vi "AdvanceWaveformPart.vi"(6 "FPGA Cycle Parameters":T1, 7 "FPGA Cycle Counters In":T2, 8 "FPGA Scan Counters In":T3 {"Current part of waveform" items=["Imaging", "Settling", "Resting"]}) -> (1 "Multiplier advance per cycle":fxp<+/-,32,0>, 2 "FPGA Cycle Counters Out":T2, 3 "FPGA Scan Counters Out":T3 {"Current part of waveform" items=["Imaging", "Settling", "Resting"]})   [LabVIEW 2010]
uses:
  FPGA_Typedefs/FPGA Scan Counters.ctl
  FPGA_Typedefs/FPGA Cycle Counters.ctl
  FPGA_Typedefs/FPGA Cycle Parameters.ctl
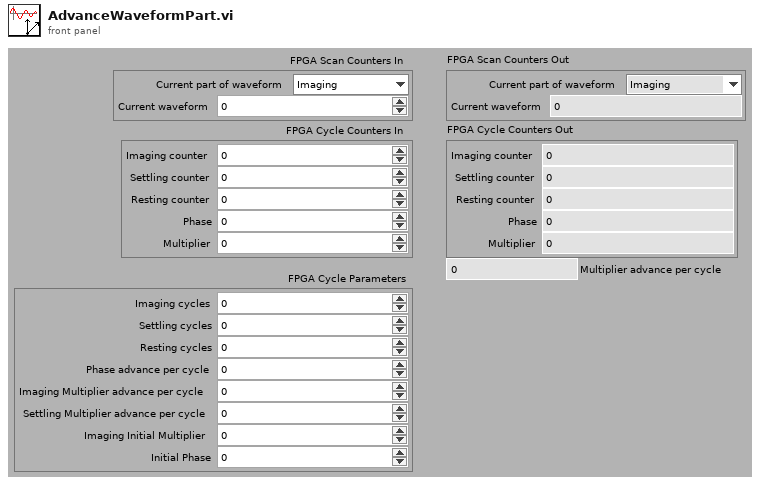
[diagram p1: front panel]
types:
  T1 = typedef "FPGA Cycle Parameters.ctl" = cluster{"Imaging cycles":i32, "Settling cycles":i32, "Resting cycles":i32, "Phase advance per cycle":fxp<+,32,0>, "Imaging Multiplier advance per cycle":fxp<+/-,32,0>, "Settling Multiplier advance per cycle":fxp<+/-,32,0>, "Imaging Initial Multiplier":fxp<+/-,43,12>, "Initial Phase":fxp<+,32,1>}
  T2 = typedef "FPGA Cycle Counters.ctl" = cluster{"Imaging counter":i32, "Settling counter":i32, "Resting counter":i32, "Phase":fxp<+,32,1>, "Multiplier":fxp<+/-,43,12>}
  T3 = typedef "FPGA Scan Counters.ctl" = cluster{"Current part of waveform":u8, "Current waveform":u16}
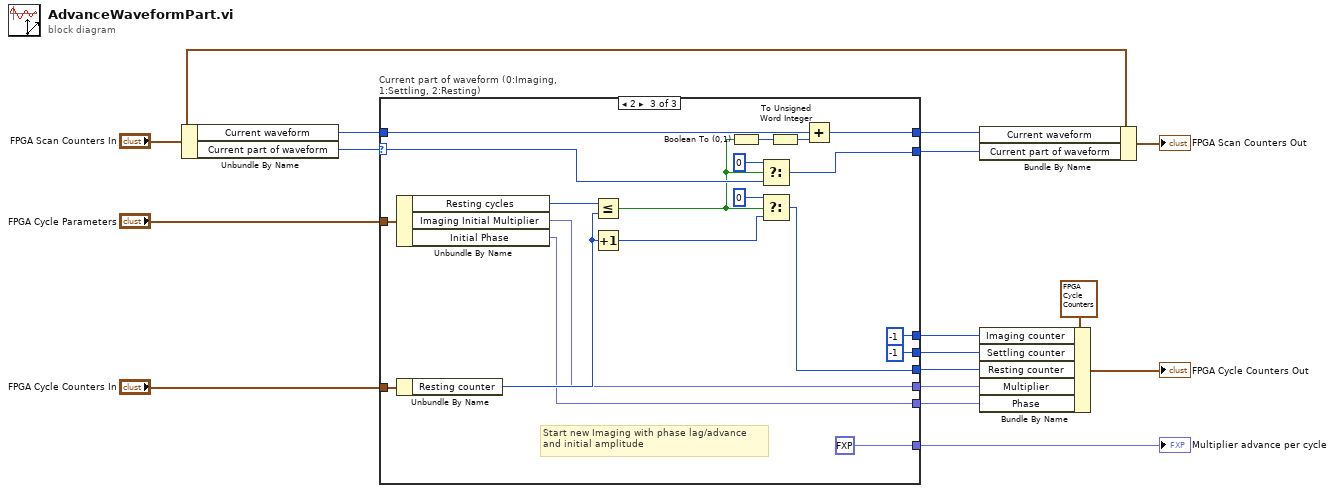
[diagram p0: block diagram]
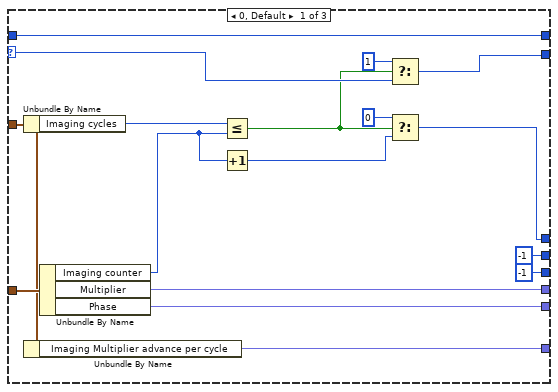
[diagram p2: hidden frame]
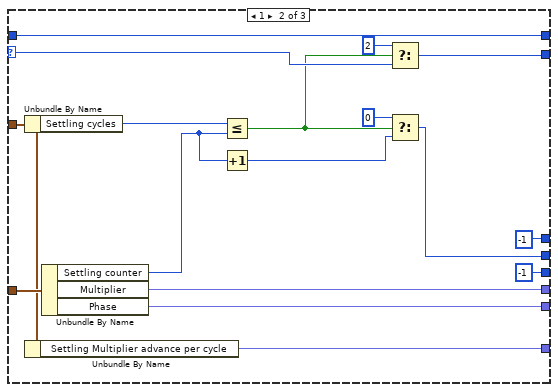
[diagram p3: hidden frame]
diagram:
  n1 = Unbundle By Name("FPGA Scan Counters In") -> ("Current waveform"=w16:u16, "Current part of waveform"=w15:u8)
  n2 = case "Current part of waveform (0:Imaging, 1:Settling, 2:Resting)" shown="2" w15 {
    selector: w15 -> [w33 w49 w69]
    tunnel: [w31 w48 w68] -> w13
    tunnel: w16 -> [w30 w47 w67]
    tunnel: [w30 w47 w66] -> w14
    tunnel: "FPGA Cycle Parameters" -> [w22 w39 w63]
    tunnel: "FPGA Cycle Counters In" -> [w29 w41 w62]
    tunnel: [w28 w43 w58] -> w11
    tunnel: [w24 w42 w57] -> w10
    tunnel: [w21 w38 fxp<+/-,32,0> 0.0 ("Settling Multiplier advance per cycle")] -> w5
    tunnel: [w17 -1 ("Imaging counter") -1 ("Imaging counter")] -> w3
    tunnel: [-1 ("t") w34 -1 ("t")] -> w2
    tunnel: [-1 ("t") -1 ("t") w53] -> w1
    frame 0, Default {
      n3 = Unbundle By Name(w22) -> ("Imaging cycles"=w27:i32)
      n4 = Unbundle By Name(w22) -> ("Imaging Multiplier advance per cycle"=w21:fxp<+/-,32,0>)
      n5 = Unbundle By Name(w29) -> ("Imaging counter"=w20:i32, "Multiplier"=w28:fxp<+/-,43,12>, "Phase"=w24:fxp<+,32,1>)
      n6 = Less Or Equal?(x=w27, y=w20) -> (x <= y?=w23:bool)
      n7 = Increment(x=w20) -> (x+1=w26:i32)
      n8 = Select(t=u8 1, s=w23, f=w33) -> (s? t:f=w31:u8)
      n9 = Select(t=0, s=w23, f=w26) -> (s? t:f=w17:i32)
    }
    frame 1 {
      n10 = Unbundle By Name(w39) -> ("Settling cycles"=w46:i32)
      n11 = Unbundle By Name(w39) -> ("Settling Multiplier advance per cycle"=w38:fxp<+/-,32,0>)
      n12 = Unbundle By Name(w41) -> ("Settling counter"=w37:i32, "Multiplier"=w43:fxp<+/-,43,12>, "Phase"=w42:fxp<+,32,1>)
      n13 = Less Or Equal?(x=w46, y=w37) -> (x <= y?=w40:bool)
      n14 = Increment(x=w37) -> (x+1=w45:i32)
      n15 = Select(t=u8 2, s=w40, f=w49) -> (s? t:f=w48:u8)
      n16 = Select(t=0, s=w40, f=w45) -> (s? t:f=w34:i32)
    }
    frame 2 {
      # "Start new Imaging with phase lag/advance\nand initial amplitude"
      n17 = Unbundle By Name(w63) -> ("Resting cycles"=w65:i32, "Imaging Initial Multiplier"=w58:fxp<+/-,43,12>, "Initial Phase"=w57:fxp<+,32,1>)
      n18 = Unbundle By Name(w62) -> ("Resting counter"=w61:i32)
      n19 = Less Or Equal?(x=w65, y=w61) -> (x <= y?=w60:bool)
      n20 = Increment(x=w61) -> (x+1=w54:i32)
      n21 = Boolean To (0,1)(Boolean=w60) -> (0, 1=w51:i16)
      n22 = Select(t=u8 0, s=w60, f=w69) -> (s? t:f=w68:u8)
      n23 = Select(t=0, s=w60, f=w54) -> (s? t:f=w53:i32)
      n24 = To Unsigned Word Integer(number=w51) -> (unsigned 16bit integer=w52:u16)
      n25 = Add(x=w67, y=w52) -> (x+y=w66:u16)
    }
  }
  "Multiplier advance per cycle" <- w5
  n26 = Bundle By Name(cluster="FPGA Scan Counters In", "Current waveform"=w14, "Current part of waveform"=w13) -> (→"FPGA Scan Counters Out":T3)
  n27 = Bundle By Name(cluster=T2 {"Imaging counter"=0, "Settling counter"=0, "Resting counter"=0, "Phase"=0.0, "Multiplier"=0.0} ("FPGA Cycle Counters Out"), "Imaging counter"=w3, "Settling counter"=w2, "Resting counter"=w1, "Multiplier"=w11, "Phase"=w10) -> (→"FPGA Cycle Counters Out":T2)
